vi "UIRef.vi"(8 "error in":errorcluster, 11 "node in":refnum<class "Device.lvclass">) -> (0 "error out":errorcluster, 2 "VI refnum":refnum<vi>, 3 "node out":refnum<class "Device.lvclass">)   [LabVIEW 2014, in "Device.lvclass"]
doc: "Stores the static reference to the UI of the node."
uses:
  Device.lvclass
  DeviceUI.vi
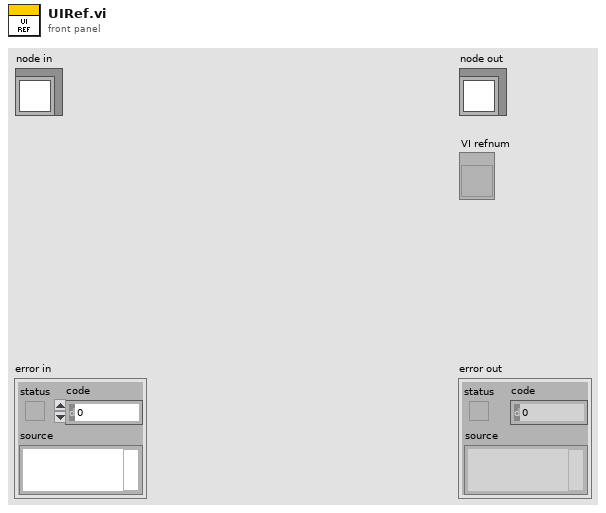
[diagram p1: front panel]
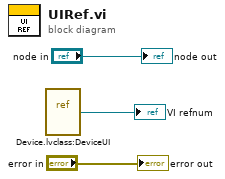
[diagram p0: block diagram]
diagram:
  n1 = vi-ref "Device.lvclass:DeviceUI.vi"() -> (→"VI refnum":refnum<vi>)
  "error out" <- "error in"
  "node out" <- "node in"
